vi "RunOperation.vi"(10 "Inputs":string[](array[string]), 11 "LUnitCLI In":refnum<class "LUnitCLI.lvclass">) -> (1 "Output/Failure":string, 2 "CLI Process Return Code":i32, 3 "LUnitCLI Out":refnum<class "LUnitCLI.lvclass">)   [LabVIEW 2020, in "LUnitCLI.lvclass"]
uses:
  LUnitCLI.lvclass
  LUnitCLI.lvclass/LUnitCLI.ctl
  <vilib>/Astemes/LUnit/Palette/API/LUnit Execution API.lvclass
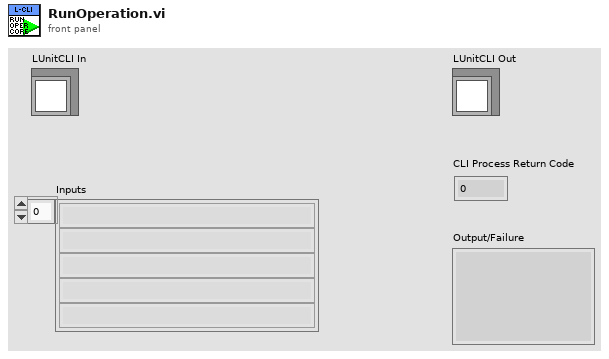
[diagram p1: front panel]
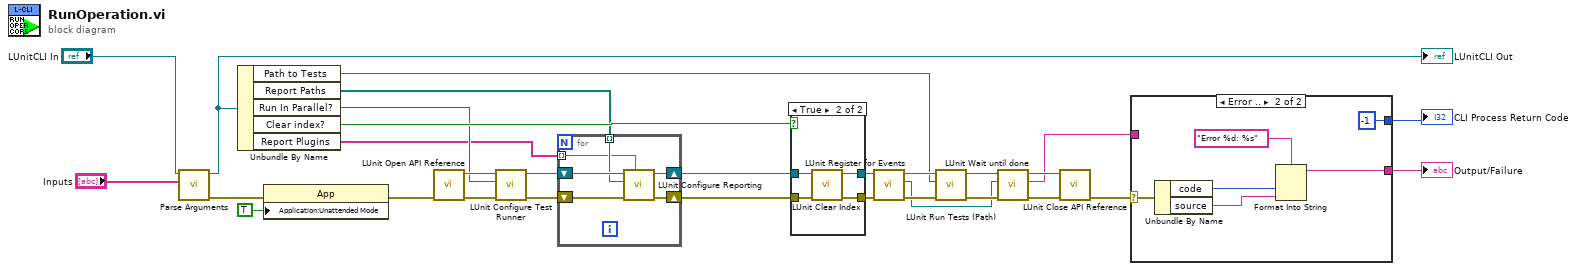
[diagram p0: block diagram]
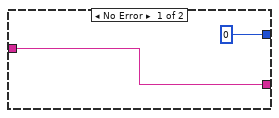
[diagram p3: hidden frame]
diagram:
  n1 = call "Parse Arguments.vi"("Inputs"="Inputs", "LUnitCLI In"="LUnitCLI In") -> ("error out"=w2:errorcluster, "LUnitCLI Out"=w26:refnum<class "LUnitCLI.lvclass">)  [unwired: 8 in]
  "LUnitCLI Out" <- w26
  n2 = Unbundle By Name(w26) -> ("Path to Tests"=w9:path, "Report Paths"=w12:path[], "Run In Parallel?"=w7:bool, "Clear index?"=w13:bool, "Report Plugins"=w4:string[])
  n3 = property class="App"(error in=w2, "Application:Unattended Mode"=TRUE) -> (error out=w1:errorcluster)  [unwired: 1 in, 1 out]
  n4 = call <vilib>:"LUnit Open API Reference.vi"("error in (no error)"=w1) -> ("error out"=w24:errorcluster, "Execution API Out"=w25:refnum<class "LUnit Execution API.lvclass">)  [unwired: 9 in]
  n5 = call <vilib>:"LUnit Configure Test Runner.vi"("error in (no error)"=w24, "Run Tests In Parallel?"=w7, "Execution API In"=w25) -> ("error out"=w22:errorcluster, "Execution API Out"=w23:refnum<class "LUnit Execution API.lvclass">)  [unwired: 7 in]
  n6 = for {
    tunnel: w12 -> [w34] mode=indexing
    shift-right: [w32] -> w5
    shift-left: w23 -> [w36]
    shift-right: [w33] -> w6
    shift-left: w22 -> [w35]
    tunnel: w4 -> [w31] mode=indexing
    n7 = call <vilib>:"LUnit Configure Reporting.vi"("Custom Reporting Plugin"=w31, "error in (no error)"=w35, "Path"=w34, "Execution API In"=w36) -> ("error out"=w33:errorcluster, "Execution API Out"=w32:refnum<class "LUnit Execution API.lvclass">)  [unwired: 6 in]
  }
  n8 = case shown="True" w13 {
    tunnel: w5 -> [w38 w42]
    tunnel: w6 -> [w37 w41]
    tunnel: [w38 w40] -> w21
    tunnel: [w37 w39] -> w20
    frame False {
    }
    frame True {
      n9 = call <vilib>:"LUnit Clear Index.vi"("error in (no error)"=w41, "Execution API In"=w42) -> ("error out"=w39:errorcluster, "Execution API Out"=w40:refnum<class "LUnit Execution API.lvclass">)  [unwired: 8 in]
    }
  }
  n10 = call <vilib>:"LUnit Register for Events.vi"("error in (no error)"=w20, "Execution API In"=w21) -> ("error out"=w18:errorcluster, "Event Registration"=w8:refnum<event-registration>, "Execution API Out"=w19:refnum<class "LUnit Execution API.lvclass">)  [unwired: 7 in]
  n11 = call <vilib>:"LUnit Run Tests (Path).vi"("error in (no error)"=w18, "Project or Class Path"=w9, "Execution API In"=w19) -> ("error out"=w16:errorcluster, "Execution API Out"=w17:refnum<class "LUnit Execution API.lvclass">)  [unwired: 7 in]
  n12 = call <vilib>:"LUnit Wait until done.vi"("error in (no error)"=w16, "Event Registration"=w8, "Execution API In"=w17) -> ("error out"=w14:errorcluster, "Output"=w11:string, "Execution API Out"=w15:refnum<class "LUnit Execution API.lvclass">)  [unwired: 6 in]
  n13 = call <vilib>:"LUnit Close API Reference.vi"("error in (no error)"=w14, "Execution API In"=w15) -> ("error out"=w10:errorcluster)  [unwired: 9 in]
  n14 = case shown="Error .." w10 {
    selector: w10 -> [_ w49]
    tunnel: [w44 w45] -> w30
    tunnel: w11 -> [w44 _]
    tunnel: [0 ("CLI Process Return Code") -1 ("CLI Process Return Code")] -> w29
    frame No Error {
    }
    frame Error {
      n15 = Unbundle By Name(w49) -> ("code"=w48:i32, "source"=w47:string)
      n16 = Format Into String(format string="Error %d: %s", w48, w47) -> (resulting string=w45:string)  [unwired: 2 in, 1 out]
    }
  }
  "CLI Process Return Code" <- w29
  "Output/Failure" <- w30
